vi "Get Host Port.vi"(11 "URI in":refnum<class "URI.lvclass">) -> (2 "Port":u16, 3 "Host":string)   [LabVIEW 2020, in "IO.lvlib" / "URI.lvclass"]
uses:
  URI.lvclass
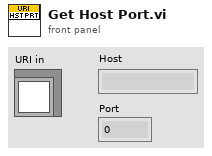
[diagram p1: front panel]
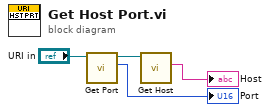
[diagram p0: block diagram]
diagram:
  n1 = call "Get Port.vi"("URI in"="URI in") -> ("Port"=→"Port":u16, "URI out"=w3:refnum<class "URI.lvclass">)  [unwired: 8 in, 1 out]
  n2 = call "Get Host.vi"("URI in"=w3) -> ("Host"=→"Host":string)  [unwired: 8 in, 2 out]
